vi "Tegam4040 -- Close4040.vi"(8 "error in (no error)":errorcluster, 11 "Instrument Session Handle":u32 format="%x") -> (0 "error out":errorcluster)   [LabVIEW 2010]
panel:
  out "VISA Error Code":i32 format="%x"
  out "Tegam Error Code":i32
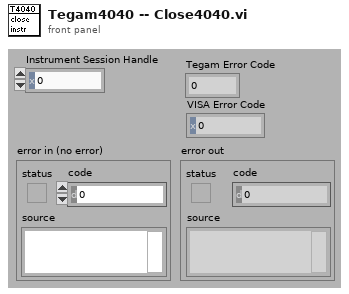
[diagram p1: front panel]
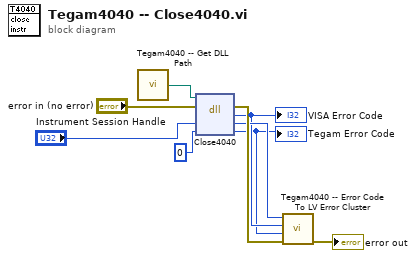
[diagram p0: block diagram]
diagram:
  n1 = call "Tegam4040 -- Get DLL Path.vi"() -> ("DLL Path"=w6:path)  [unwired: 8 in]
  n2 = dll-call lib="C:/Documents and Settings/Administrator/My Documents/Visual Studio 2005/Projects/Tegam4040CDriver/debug/Tegam4040CDriver.dll" fn="Close4040"(path in=w6, error in="error in (no error)", "instrSession"="Instrument Session Handle", "tegamError"=0) -> (error out=w8:errorcluster, "status"=w2:i32, "instrSession"=w3:u32, "tegamError"=w1:i32)  [unwired: 1 in, 1 out]
  "Tegam Error Code" <- w1
  "VISA Error Code" <- w2
  n3 = call "Tegam4040 -- Error Code To LV Error Cluster.vi"("error in (no error)"=w8, "Driver Error Code"=w1, "VISA Error Code"=w2, "Instrument Session Handle"=w3) -> ("error out"=→"error out":errorcluster)  [unwired: 7 in]
